vi "Build Init Request.vi"(6 "resource":string, 7 "connect timeout":dbl, 8 "error in (no error)":errorcluster, 9 "slsc type":T1, 10 "reservation access":i32, 11 "reservation group":string) -> (0 "error out":errorcluster, 3 "JSON Tree out (JSON Object)":variant)   [LabVIEW 2016, in "SLSC Interfaces.lvlib" / "SLSC Remote.lvclass"]
uses:
  SLSC Remote.lvclass
  SLSC Interface Class/slsc type.ctl
  <vilib>/rajsite/i3-json/JSON Generation/Create Value Files/Create Value - Object.vi
  <vilib>/rajsite/i3-json/JSON Generation/Add Object Parameter Files/Add Object Parameter - String.vi
  <vilib>/rajsite/i3-json/JSON Generation/Add Object Parameter Files/Add Object Parameter - Numeric.vi
  <vilib>/rajsite/i3-json/i3-json.lvlib
  SLSC Interface Class/SLSC Interface.lvclass
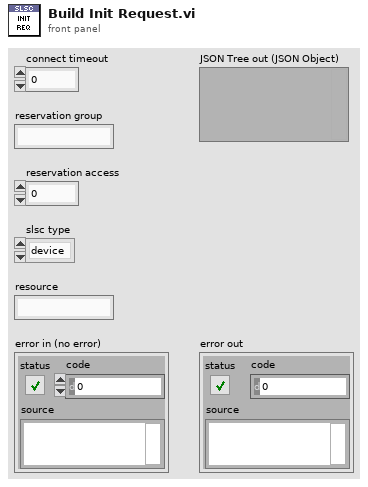
[diagram p1: front panel]
types:
  T1 = typedef "SLSC Interfaces.lvlib/SLSC Interface.lvclass/slsc type.ctl" = enum16{"device", "nvmem", "channel", "none"}
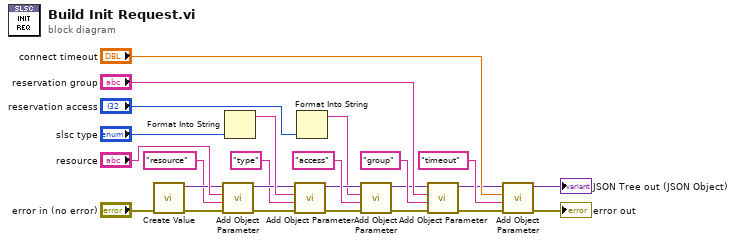
[diagram p0: block diagram]
diagram:
  n1 = call-poly <vilib>:"Create Value.vi"("error in (no error)"="error in (no error)") -> ("error out"=w5:errorcluster, "JSON Tree"=w8:variant)  [unwired: 9 in]
  n2 = call-poly <vilib>:"Add Object Parameter.vi"("error in (no error)"=w5, "Name"="resource", "String"="resource", "JSON Tree in (JSON Object)"=w8) -> ("error out"=w6:errorcluster, "JSON Tree out (JSON Object)"=w7:variant)  [unwired: 6 in]
  n3 = Format Into String("slsc type") -> (resulting string=w9:string)  [unwired: 3 in, 1 out]
  n4 = call-poly <vilib>:"Add Object Parameter.vi"("error in (no error)"=w6, "Name"="type", "String"=w9, "JSON Tree in (JSON Object)"=w7) -> ("error out"=w13:errorcluster, "JSON Tree out (JSON Object)"=w14:variant)  [unwired: 6 in]
  n5 = Format Into String("reservation access") -> (resulting string=w1:string)  [unwired: 3 in, 1 out]
  n6 = call-poly <vilib>:"Add Object Parameter.vi"("error in (no error)"=w13, "Name"="access", "String"=w1, "JSON Tree in (JSON Object)"=w14) -> ("error out"=w17:errorcluster, "JSON Tree out (JSON Object)"=w16:variant)  [unwired: 6 in]
  n7 = call-poly <vilib>:"Add Object Parameter.vi"("error in (no error)"=w17, "Name"="group", "String"="reservation group", "JSON Tree in (JSON Object)"=w16) -> ("error out"=w21:errorcluster, "JSON Tree out (JSON Object)"=w20:variant)  [unwired: 6 in]
  n8 = call-poly <vilib>:"Add Object Parameter.vi"("error in (no error)"=w21, "Name"="timeout", "Numeric"="connect timeout", "JSON Tree in (JSON Object)"=w20) -> ("error out"=→"error out":errorcluster, "JSON Tree out (JSON Object)"=→"JSON Tree out (JSON Object)":variant)  [unwired: 6 in]
